vi "Balance Movement.vi"(7 "Value":u16, 8 "error out 2":errorcluster, 9 "Speed":dbl, 10 "Move":T1(ring), 11 "FPGA VI Reference Out":refnum<k20>) -> (0 "error out":errorcluster, 2 "STOP NOW":bool, 3 "FPGA VI Reference Out 2":refnum<k20>)   [LabVIEW 2019]
uses:
  <vilib>/Platform/TimedLoop/XDataNode/timing_clust.ctl
  <vilib>/Platform/TimedLoop/XDataNode/nitl_modes.ctl
  <vilib>/Platform/TimedLoop/XDataNode/wakeup.ctl
  <vilib>/robotics/Steering/Mecanum Wheel/Roller Orientation.ctl
  <vilib>/robotics/Steering/Wheel/Wheel Parameters.ctl
  <vilib>/robotics/Steering/Wheel/Rotation Direction.ctl
  <vilib>/robotics/Steering/Mecanum Steering Frame/NI_Robotics_Mecanum Steering Frame.lvclass
  C:/Program Files (x86)/National Instruments/LabVIEW 2019/vi.lib/robotics/Steering/Steering Frame/NI_Robotics_Steering Frame.lvclass
  <vilib>/robotics/Steering/Mecanum Wheel/Create Mecanum Wheel.vi
  <vilib>/robotics/Steering/Mecanum Steering Frame/Create Mecanum Steering Frame.vi
  <vilib>/Utility/error.llb/Error Cluster From Error Code.vi
  <vilib>/rvi/errors/niLvFpgaAdjustHostInterfaceError.vi
  <vilib>/robotics/Steering/Steering Frame/Apply Steering Frame Velocity to Motors.vi
  <vilib>/platform/TimedLoop/XDataNode/XDataNode.xnode
  <vilib>/robotics/Steering/Create Steering Frame/NI_Robotics_Create Steering Frame.xnode
  <vilib>/robotics/Steering/Class Type Definitions/Mecanum Steering Frame.ctl
  <vilib>/rvi/interface/nirviReadWriteControl/nirviReadWriteControl.xnode
  <vilib>/rvi/interface/Simulation/niFpgaSimulationCallBeginRW.vi
  <vilib>/Platform/TimedLoop/XDataNode/XDNodeRunTimeDep.lvlib
  <vilib>/robotics/Steering/Class Type Definitions/NI_Robotics_Steering Class Types.lvlib
  <vilib>/robotics/Steering/Mecanum Wheel/NI_Robotics_Mecanum Wheel.lvclass
  <vilib>/robotics/Steering/Wheel/NI_Robotics_Wheel.lvclass
  <vilib>/robotics/Steering/Steering Frame/NI_Robotics_Steering Frame.lvclass
  NiFpgaLv.dll
  C:/Program Files (x86)/National Instruments/LabVIEW 2019/vi.lib/robotics/Steering/Special Steering Frame/NI_Robotics_Special Steering Frame.lvclass
panel:
  out "IR 1":u16
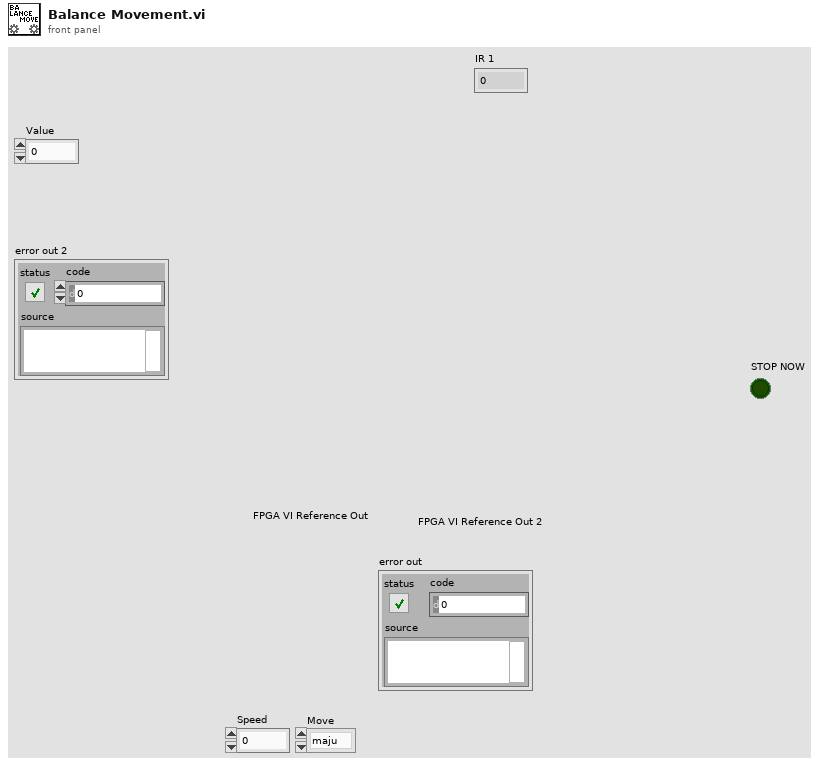
[diagram p1: front panel]
types:
  T1 = enum16{"maju", "mundur", "kanan", "kiri", "atas kanan", "atas kiri", "bawah kanan", "bawah kiri", "putar kanan", "putar kiri"}
  T2 = typedef "NI_Robotics_Steering Class Types.lvlib/Mecanum Steering Frame.ctl" = refnum<class "NI_Robotics_Mecanum Steering Frame.lvclass">
  T3 = typedef "XDNodeRunTimeDep.lvlib/timing_clust.ctl" = cluster{"Expected End [f-1]":u64, "Actual End [f-1]":u64, "Finished Late? [f-1]":bool, "Expected End [i-1]":u64, "Actual End [i-1]":u64, "Finished Late? [i-1]":bool, "Expected Start [i]":u64, "Actual Start [i]":u64, "Expected Start [f]":u64, "Actual Start [f]":u64, "Source Name":string, "Structure Name":string, "Period":i64, "Deadline":i64, "Offset":i64, "Start":i64, "Priority":i32, "Timeout":i32, "Mode":T4, "Wakeup Reason":T5, "Error":errorcluster, "Source Type":string, "Secondary Source Type":string, "Global End Time":u64, "Global Start Time":u64, "Frame Duration":u64, "Iteration Duration":u64, "Assigned CPU":i32, "I/O Scan Engine Mode":u32}
  T4 = typedef "XDNodeRunTimeDep.lvlib/nitl_modes.ctl" = enum32{"No Change", "Process missed periods, maintain original phase", "Discard missed periods, maintain original phase", "Process missed periods, ignore original phase", "Discard missed periods, ignore original phase"}
  T5 = typedef "XDNodeRunTimeDep.lvlib/wakeup.ctl" = enum32{"Normal", "Aborted", "Asynchronous wakeup", "Timing source error", "Timed loop error", "Timeout"}
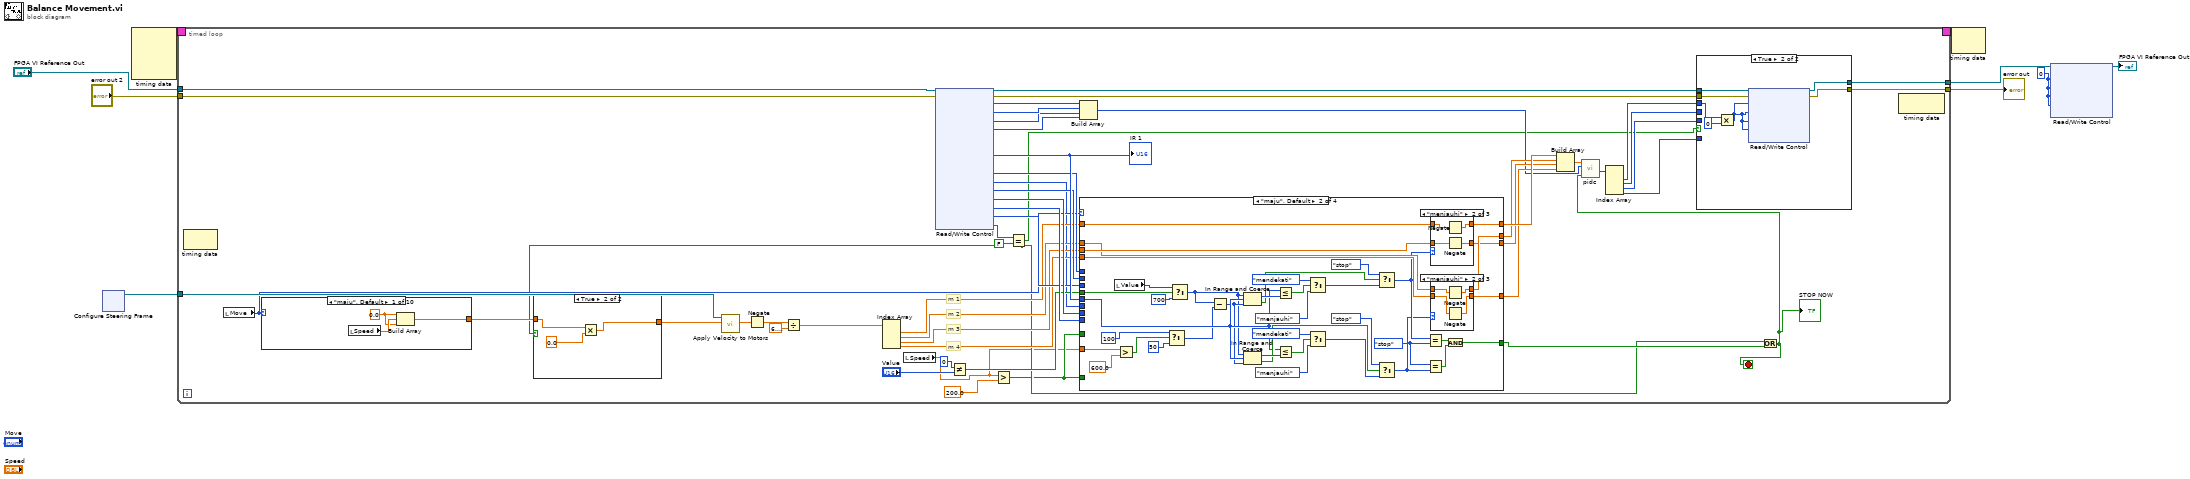
[diagram p0: block diagram]
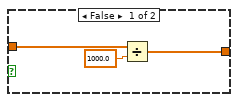
[diagram p2: hidden frame]
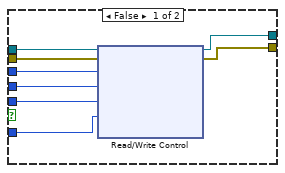
[diagram p3: hidden frame]
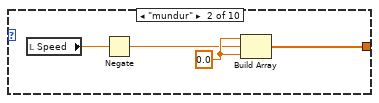
[diagram p4: hidden frame]
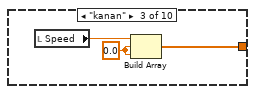
[diagram p5: hidden frame]
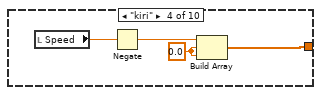
[diagram p6: hidden frame]
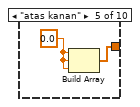
[diagram p7: hidden frame]
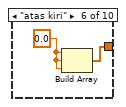
[diagram p8: hidden frame]
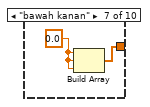
[diagram p9: hidden frame]
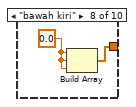
[diagram p10: hidden frame]
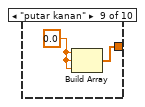
[diagram p11: hidden frame]
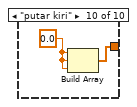
[diagram p12: hidden frame]
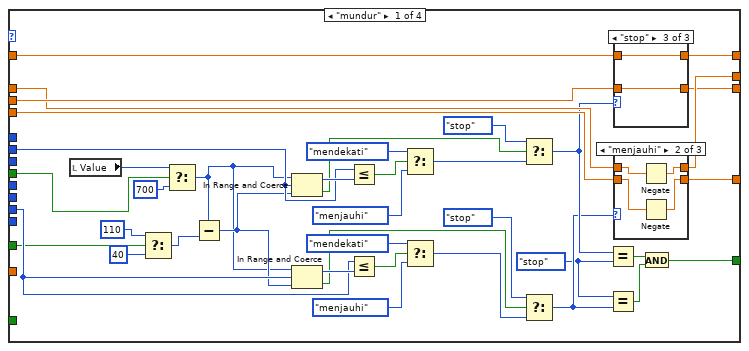
[diagram p13: hidden frame]
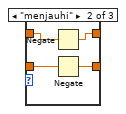
[diagram p17: hidden frame]
diagram:
  w2 = i16 0 ("M1")
  n1 = xnode ("Configure Steering Frame")() -> ("mecanum steering frame out"=w5:T2)  [unwired: 1 in, 1 out]
  n2 = node-c288() -> (w7:T3)  [unwired: 4 in]
  n3 = timed-loop {
    timing: w7 -> [_]
    timing-out: [_] -> w6
    tunnel: "FPGA VI Reference Out" -> [w60]
    tunnel: "error out 2" -> [w56]
    tunnel: [w59] -> w8
    tunnel: [w58] -> w9
    tunnel: w5 -> [w54]
    stop <- w13 stop-if-true
    # "m 4"
    # "m 3"
    # "m 2"
    # "m 1"
    n4 = node-c288() -> ()  [unwired: 1 in, 1 out]
    n5 = local read "Move"() -> (w26:T1)
    n6 = case shown="\"maju\", Default" w26 {
      tunnel: [w82 w86 w90 w94 w97 w99 w101 w103 w105 w107] -> w27
      frame "maju", Default {
        w83 = 0.0 ("element")
        n7 = local read "Speed"() -> (w84:dbl)
        n8 = Build Array(w83, w84, w83) -> (w82:dbl[])
      }
      frame "mundur" {
        w87 = 0.0 ("element")
        n9 = local read "Speed"() -> (w88:dbl)
        n10 = Negate(x=w88) -> (-x=w85:dbl)
        n11 = Build Array(w87, w85, w87) -> (w86:dbl[])
      }
      frame "kanan" {
        w89 = 0.0 ("element")
        n12 = local read "Speed"() -> (w91:dbl)
        n13 = Build Array(w91, w89, w89) -> (w90:dbl[])
      }
      frame "kiri" {
        w92 = 0.0 ("element")
        n14 = local read "Speed"() -> (w95:dbl)
        n15 = Negate(x=w95) -> (-x=w93:dbl)
        n16 = Build Array(w93, w92, w92) -> (w94:dbl[])
      }
      frame "atas kanan" {
        w96 = 0.0 ("element")
        n17 = Build Array(w96, w96, w96) -> (w97:dbl[])
      }
      frame "atas kiri" {
        w98 = 0.0 ("element")
        n18 = Build Array(w98, w98, w98) -> (w99:dbl[])
      }
      frame "bawah kanan" {
        w100 = 0.0 ("element")
        n19 = Build Array(w100, w100, w100) -> (w101:dbl[])
      }
      frame "bawah kiri" {
        w102 = 0.0 ("element")
        n20 = Build Array(w102, w102, w102) -> (w103:dbl[])
      }
      frame "putar kanan" {
        w104 = 0.0 ("element")
        n21 = Build Array(w104, w104, w104) -> (w105:dbl[])
      }
      frame "putar kiri" {
        w106 = 0.0 ("element")
        n22 = Build Array(w106, w106, w106) -> (w107:dbl[])
      }
    }
    n23 = local read "Speed"() -> (w10:dbl)
    n24 = xnode "Read/Write Control"("FPGA VI Reference In"=w60, "error in"=w56) -> ("FPGA VI Reference Out"=w57:refnum<k20>, "error out"=w55:errorcluster, "ENC M1"=w51:i32, "ENC M2"=w50:i32, "ENC M3"=w49:i32, "ENC M4"=w48:i32, "IR 1"=w41:u16, "IR 3"=w40:u16, "IR 4"=w18:u16, "IR 5"=w39:u16, "IR 6"=w38:u16, "IR 7"=w37:u16, "IR 8"=w36:u16, "START BUTTON"=w16:bool)  [unwired: 3 out]
    "IR 1" <- w41
    n25 = Not Equal?(x=u16 0, y="Value") -> (x != y?=w19:bool)
    n26 = Greater?(x=w10, y=200.0) -> (0:w12:bool)
    n27 = Equal?(x=w16, y=FALSE) -> (x = y?=w14:bool)
    n28 = case shown="True" w14 {
      tunnel: w27 -> [w63 w66]
      tunnel: [w62 w65] -> w22
      frame False {
        n29 = Divide(x=w63, y=1000.0) -> (x/y=w62:dbl[])
      }
      frame True {
        n30 = Multiply(x=w66, y=0.0) -> (x*y=w65:dbl[])
      }
    }
    n31 = call-poly <vilib>:"Apply Velocity to Motors.vi"("steering frame velocity"=w22, "steering frame in"=w54) -> ("ccw motor velocity setpoints"=w52:dbl[])  [unwired: 5 in, 4 out]
    n32 = Negate(x=w52) -> (-x=w53:dbl[])
    n33 = Divide(x=w53, y=6.283185307179586) -> (x/y=w43:dbl[])
    n34 = Index Array(array=w43) -> (element #1=w35:dbl, element #2=w34:dbl, element #3=w33:dbl, element #4=w32:dbl)  [unwired: 4 in]
    n35 = Build Array(w51, w50, w49, w48) -> (w24:i32[])
    n36 = case shown="\"maju\", Default" w26 {
      tunnel: w41 -> [_ w181 _ _]
      tunnel: w40 -> [_ _ _ w277]
      tunnel: w18 -> [_ _ _ w276]
      tunnel: w39 -> [w114 _ _ _]
      tunnel: w38 -> [w115 _ _ _]
      tunnel: w37 -> [_ _ w223 _]
      tunnel: w36 -> [_ _ w224 _]
      tunnel: w35 -> [w134 w189 w243 w298]
      tunnel: w34 -> [w132 w187 w242 w297]
      tunnel: w33 -> [w133 w188 w241 w296]
      tunnel: w32 -> [w131 w186 w240 w295]
      tunnel: [w127 w182 w239 w294] -> w31
      tunnel: [w129 w184 w238 w293] -> w30
      tunnel: [w128 w183 w237 w292] -> w29
      tunnel: [w130 w185 w236 w291] -> w28
      tunnel: [w120 w175 w233 w285] -> w17
      tunnel: w19 -> [w116 w170 w225 w278]
      tunnel: w12 -> [_ _ w222 w275]
      tunnel: w12 -> [w111 _ _ _]
      tunnel: w10 -> [_ w168 _ _]
      frame "mundur" {
        w119 = enum16{"mendekati", "menjauhi", "stop", "start"}."stop" ("t")
        n37 = local read "Value"() -> (w118:u16)
        n38 = Select(t=u16 110 ("f"), s=w111, f=u16 40) -> (s? t:f=w108:u16)
        n39 = Select(t=w118, s=w116, f=u16 700) -> (s? t:f=w112:u16)
        n40 = Subtract(x=w112, y=w108) -> (x-y=w113:u16)
        n41 = In Range and Coerce(upper limit=w112, x=w114, lower limit=w113) -> (coerced(x)=w146:u16, In Range?=w141:bool)
        n42 = In Range and Coerce(upper limit=w112, x=w115, lower limit=w113) -> (coerced(x)=w140:u16, In Range?=w135:bool)
        n43 = Less Or Equal?(x=w114, y=w146) -> (x <= y?=w142:bool)
        n44 = Less Or Equal?(x=w115, y=w140) -> (x <= y?=w136:bool)
        n45 = Select(t=enum16{"mendekati", "menjauhi", "stop", "start"}."mendekati", s=w142, f=enum16{"mendekati", "menjauhi", "stop", "start"}."menjauhi") -> (s? t:f=w144:enum16{"mendekati", "menjauhi", "stop", "start"})
        n46 = Select(t=enum16{"mendekati", "menjauhi", "stop", "start"}."mendekati", s=w136, f=enum16{"mendekati", "menjauhi", "stop", "start"}."menjauhi") -> (s? t:f=w138:enum16{"mendekati", "menjauhi", "stop", "start"})
        n47 = Select(t=enum16{"mendekati", "menjauhi", "stop", "start"}."stop", s=w141, f=w144) -> (s? t:f=w122:enum16{"mendekati", "menjauhi", "stop", "start"})
        n48 = Select(t=enum16{"mendekati", "menjauhi", "stop", "start"}."stop", s=w135, f=w138) -> (s? t:f=w121:enum16{"mendekati", "menjauhi", "stop", "start"})
        n49 = Equal?(x=w122, y=w119) -> (x = y?=w126:bool)
        n50 = Equal?(x=w119, y=w121) -> (x = y?=w125:bool)
        n51 = case shown="\"stop\"" w122 {
          tunnel: w134 -> [w156 w160 w162]
          tunnel: w133 -> [w155 w158 w161]
          tunnel: [w156 w159 w162] -> w127
          tunnel: [w155 w157 w161] -> w128
          frame "mendekati", Default {
          }
          frame "menjauhi" {
            n52 = Negate(x=w160) -> (-x=w159:dbl)
            n53 = Negate(x=w158) -> (-x=w157:dbl)
          }
          frame "stop" {
          }
        }
        n54 = case shown="\"menjauhi\"" w121 {
          tunnel: w132 -> [w148 w152 w154]
          tunnel: w131 -> [w147 w151 w153]
          tunnel: [w147 w150 w153] -> w130
          tunnel: [w148 w149 w154] -> w129
          frame "mendekati", Default {
          }
          frame "menjauhi" {
            n55 = Negate(x=w152) -> (-x=w149:dbl)
            n56 = Negate(x=w151) -> (-x=w150:dbl)
          }
          frame "stop" {
          }
        }
        n57 = And(x=w126, y=w125) -> (x .and. y?=w120:bool)
      }
      frame "maju", Default {
        w176 = enum16{"mendekati", "menjauhi", "stop", "start"}."stop" ("t")
        n58 = local read "Value"() -> (w173:u16)
        n59 = Greater?(x=w168, y=600.0) -> (0:w166:bool)
        n60 = Select(t=u16 100 ("x"), s=w166, f=u16 50 ("x")) -> (s? t:f=w163:u16)
        n61 = Select(t=w173, s=w170, f=u16 700) -> (s? t:f=w169:u16)
        n62 = Subtract(x=w169, y=w163) -> (x-y=w171:u16)
        n63 = In Range and Coerce(upper limit=w169, x=w181, lower limit=w171) -> (coerced(x)=w202:u16, In Range?=w174:bool)
        n64 = In Range and Coerce(upper limit=w169, x=w181, lower limit=w171) -> (coerced(x)=w196:u16, In Range?=w190:bool)
        n65 = Less Or Equal?(x=w181, y=w202) -> (x <= y?=w197:bool)
        n66 = Less Or Equal?(x=w181, y=w196) -> (x <= y?=w191:bool)
        n67 = Select(t=enum16{"mendekati", "menjauhi", "stop", "start"}."mendekati", s=w197, f=enum16{"mendekati", "menjauhi", "stop", "start"}."menjauhi") -> (s? t:f=w200:enum16{"mendekati", "menjauhi", "stop", "start"})
        n68 = Select(t=enum16{"mendekati", "menjauhi", "stop", "start"}."mendekati", s=w191, f=enum16{"mendekati", "menjauhi", "stop", "start"}."menjauhi") -> (s? t:f=w194:enum16{"mendekati", "menjauhi", "stop", "start"})
        n69 = Select(t=enum16{"mendekati", "menjauhi", "stop", "start"}."stop", s=w174, f=w200) -> (s? t:f=w178:enum16{"mendekati", "menjauhi", "stop", "start"})
        n70 = Select(t=enum16{"mendekati", "menjauhi", "stop", "start"}."stop", s=w190, f=w194) -> (s? t:f=w177:enum16{"mendekati", "menjauhi", "stop", "start"})
        n71 = Equal?(x=w178, y=w176) -> (x = y?=w180:bool)
        n72 = Equal?(x=w176, y=w177) -> (x = y?=w179:bool)
        n73 = case shown="\"menjauhi\"" w178 {
          tunnel: w189 -> [w212 w216 w218]
          tunnel: w188 -> [w211 w214 w217]
          tunnel: [w212 w215 w218] -> w182
          tunnel: [w211 w213 w217] -> w183
          frame "mendekati", Default {
          }
          frame "menjauhi" {
            n74 = Negate(x=w216) -> (-x=w215:dbl)
            n75 = Negate(x=w214) -> (-x=w213:dbl)
          }
          frame "stop" {
          }
        }
        n76 = case shown="\"menjauhi\"" w177 {
          tunnel: w187 -> [w204 w208 w210]
          tunnel: w186 -> [w203 w207 w209]
          tunnel: [w203 w206 w209] -> w185
          tunnel: [w204 w205 w210] -> w184
          frame "mendekati", Default {
          }
          frame "menjauhi" {
            n77 = Negate(x=w208) -> (-x=w205:dbl)
            n78 = Negate(x=w207) -> (-x=w206:dbl)
          }
          frame "stop" {
          }
        }
        n79 = And(x=w180, y=w179) -> (x .and. y?=w175:bool)
      }
      frame "kanan" {
        w230 = enum16{"mendekati", "menjauhi", "stop", "start"}."stop" ("t")
        n80 = local read "Value"() -> (w229:u16)
        n81 = Select(t=u16 110, s=w222, f=u16 50 ("y")) -> (s? t:f=w219:u16)
        n82 = Select(t=w229, s=w225, f=u16 1100) -> (s? t:f=w226:u16)
        n83 = Subtract(x=w226, y=w219) -> (x-y=w227:u16)
        n84 = In Range and Coerce(upper limit=w226, x=w224, lower limit=w227) -> (coerced(x)=w257:u16, In Range?=w251:bool)
        n85 = In Range and Coerce(upper limit=w226, x=w223, lower limit=w227) -> (coerced(x)=w250:u16, In Range?=w244:bool)
        n86 = Less Or Equal?(x=w224, y=w257) -> (x <= y?=w252:bool)
        n87 = Less Or Equal?(x=w223, y=w250) -> (x <= y?=w245:bool)
        n88 = Select(t=enum16{"mendekati", "menjauhi", "stop", "start"}."mendekati", s=w252, f=enum16{"mendekati", "menjauhi", "stop", "start"}."menjauhi") -> (s? t:f=w255:enum16{"mendekati", "menjauhi", "stop", "start"})
        n89 = Select(t=enum16{"mendekati", "menjauhi", "stop", "start"}."mendekati", s=w245, f=enum16{"mendekati", "menjauhi", "stop", "start"}."menjauhi") -> (s? t:f=w248:enum16{"mendekati", "menjauhi", "stop", "start"})
        n90 = Select(t=enum16{"mendekati", "menjauhi", "stop", "start"}."stop", s=w251, f=w255) -> (s? t:f=w232:enum16{"mendekati", "menjauhi", "stop", "start"})
        n91 = Select(t=enum16{"mendekati", "menjauhi", "stop", "start"}."stop", s=w244, f=w248) -> (s? t:f=w231:enum16{"mendekati", "menjauhi", "stop", "start"})
        n92 = Equal?(x=w232, y=w230) -> (x = y?=w235:bool)
        n93 = Equal?(x=w230, y=w231) -> (x = y?=w234:bool)
        n94 = case shown="\"mendekati\", Default" w232 {
          tunnel: w243 -> [w266 w270 _]
          tunnel: w242 -> [w265 w268 _]
          tunnel: [w266 w269 w271] -> w239
          tunnel: [w265 w267 w271] -> w238
          frame "mendekati", Default {
          }
          frame "menjauhi" {
            n95 = Negate(x=w270) -> (-x=w269:dbl)
            n96 = Negate(x=w268) -> (-x=w267:dbl)
          }
          frame "stop" {
            w271 = 0.0
          }
        }
        n97 = case shown="\"menjauhi\"" w231 {
          tunnel: w241 -> [w259 w263 _]
          tunnel: w240 -> [w258 w262 _]
          tunnel: [w258 w261 w264] -> w236
          tunnel: [w259 w260 w264] -> w237
          frame "mendekati", Default {
          }
          frame "menjauhi" {
            n98 = Negate(x=w263) -> (-x=w260:dbl)
            n99 = Negate(x=w262) -> (-x=w261:dbl)
          }
          frame "stop" {
            w264 = 0.0
          }
        }
        n100 = And(x=w235, y=w234) -> (x .and. y?=w233:bool)
      }
      frame "kiri" {
        w288 = enum16{"mendekati", "menjauhi", "stop", "start"}."stop" ("t")
        n101 = local read "Value"() -> (w282:u16)
        n102 = Select(t=w282, s=w278, f=u16 1100) -> (s? t:f=w279:u16)
        n103 = Select(t=u16 110, s=w275, f=u16 75 ("y")) -> (s? t:f=w272:u16)
        n104 = Subtract(x=w279, y=w272) -> (x-y=w280:u16)
        n105 = In Range and Coerce(upper limit=w279, x=w277, lower limit=w280) -> (coerced(x)=w310:u16, In Range?=w305:bool)
        n106 = In Range and Coerce(upper limit=w279, x=w276, lower limit=w280) -> (coerced(x)=w304:u16, In Range?=w299:bool)
        n107 = Less Or Equal?(x=w277, y=w310) -> (x <= y?=w306:bool)
        n108 = Less Or Equal?(x=w276, y=w304) -> (x <= y?=w300:bool)
        n109 = Select(t=enum16{"mendekati", "menjauhi", "stop", "start"}."mendekati", s=w306, f=enum16{"mendekati", "menjauhi", "stop", "start"}."menjauhi") -> (s? t:f=w308:enum16{"mendekati", "menjauhi", "stop", "start"})
        n110 = Select(t=enum16{"mendekati", "menjauhi", "stop", "start"}."mendekati", s=w300, f=enum16{"mendekati", "menjauhi", "stop", "start"}."menjauhi") -> (s? t:f=w302:enum16{"mendekati", "menjauhi", "stop", "start"})
        n111 = Select(t=enum16{"mendekati", "menjauhi", "stop", "start"}."stop", s=w305, f=w308) -> (s? t:f=w284:enum16{"mendekati", "menjauhi", "stop", "start"})
        n112 = Select(t=enum16{"mendekati", "menjauhi", "stop", "start"}."stop", s=w299, f=w302) -> (s? t:f=w283:enum16{"mendekati", "menjauhi", "stop", "start"})
        n113 = Equal?(x=w284, y=w288) -> (x = y?=w287:bool)
        n114 = Equal?(x=w283, y=w288) -> (x = y?=w286:bool)
        n115 = case shown="\"menjauhi\"" w284 {
          tunnel: w298 -> [w319 w323 _]
          tunnel: w297 -> [w318 w321 _]
          tunnel: [w319 w322 w324] -> w294
          tunnel: [w318 w320 w324] -> w293
          frame "mendekati", Default {
          }
          frame "menjauhi" {
            n116 = Negate(x=w323) -> (-x=w322:dbl)
            n117 = Negate(x=w321) -> (-x=w320:dbl)
          }
          frame "stop" {
            w324 = 0.0
          }
        }
        n118 = case shown="\"menjauhi\"" w283 {
          tunnel: w296 -> [w312 w316 _]
          tunnel: w295 -> [w311 w315 _]
          tunnel: [w311 w314 w317] -> w291
          tunnel: [w312 w313 w317] -> w292
          frame "mendekati", Default {
          }
          frame "menjauhi" {
            n119 = Negate(x=w316) -> (-x=w313:dbl)
            n120 = Negate(x=w315) -> (-x=w314:dbl)
          }
          frame "stop" {
            w317 = 0.0
          }
        }
        n121 = And(x=w287, y=w286) -> (x .and. y?=w285:bool)
      }
    }
    n122 = Build Array(w31, w30, w29, w28) -> (w25:dbl[])
    n123 = Or(x=w14, y=w17) -> (x .or. y?=w13:bool)
    "STOP NOW" <- w13
    n124 = call "pidc.vi"("Stop"=w13, "input encoder 2"=w24, "input rps"=w25) -> ("Output duty cycle"=w23:i16[])  [unwired: 8 in]
    n125 = Index Array(array=w23) -> (element #1=w47:i16, element #2=w46:i16, element #3=w45:i16, element #4=w44:i16)  [unwired: 4 in]
    n126 = case shown="True" w14 {
      tunnel: [w74 w81] -> w59
      tunnel: [w73 w80] -> w58
      tunnel: w57 -> [w72 w79]
      tunnel: w55 -> [w71 w78]
      tunnel: w47 -> [w70 w77]
      tunnel: w46 -> [w69 _]
      tunnel: w45 -> [w68 _]
      tunnel: w44 -> [w67 _]
      frame False {
        n127 = xnode "Read/Write Control"("FPGA VI Reference In"=w72, "error in"=w71, "M1"=w70, "M2"=w69, "M3"=w68, "M4"=w67) -> ("FPGA VI Reference Out"=w74:refnum<k20>, "error out"=w73:errorcluster)  [unwired: 1 in]
      }
      frame True {
        n128 = Multiply(x=w77, y=i16 0) -> (x*y=w75:i16)
        n129 = xnode "Read/Write Control"("FPGA VI Reference In"=w79, "error in"=w78, "M1"=w75, "M2"=w75, "M3"=w75, "M4"=w75) -> ("FPGA VI Reference Out"=w81:refnum<k20>, "error out"=w80:errorcluster)  [unwired: 1 in]
      }
    }
    n130 = node-c288() -> ()  [unwired: 1 in, 1 out]
  }
  "error out" <- w9
  n131 = node-c288(w6) -> ()  [unwired: 1 out]
  n132 = xnode "Read/Write Control"("FPGA VI Reference In"=w8, "M1"=w2, "M2"=w2, "M3"=w2, "M4"=w2) -> ("FPGA VI Reference Out"=→"FPGA VI Reference Out 2":refnum<k20>)  [unwired: 2 in, 1 out]
